vi "LoadData.vi"(8 "error in (no error)":errorcluster, 11 "AllData In":T1 {"FlukeData"."DataAnalysisArray"."TimeStamp" format="%^<%.3X\n%x>T"; "FlukeData"."ModelDataArray"."FREQUENCY" format="%#_6f"; "FlukeData"."ModelDataArray"."TimeStamp" format="%^<%.3X\n%x>T"; "FlukeData"."PMUDataArray"."FREQUENCY" format="%#_6f"; "FlukeData"."PMUDataArray"."TimeStamp" format="%^<%.3X\n%x>T"; "NISTData"."DataAnlysisArray"."Time" format="%.6f"; "NISTData"."DataAnlysisArray"."TimeStamp" format="%^<%.3X\n%x>T"; "NISTData"."DUTDataArray"."TimeStamp" format="%^<%.3X\n%x>T"; "NISTData"."DUTDataArray"."Time" format="%.6f"; "NISTData"."NIDataArray"."TimeStamp" format="%^<%.3X\n%x>T"; "NISTData"."NIDataArray"."Time" format="%.6f"}) -> (0 "error out":errorcluster, 3 "AllData Out":T1 {"FlukeData"."DataAnalysisArray"."TimeStamp" format="%^<%.3X\n%x>T"; "FlukeData"."ModelDataArray"."FREQUENCY" format="%#_6f"; "FlukeData"."ModelDataArray"."TimeStamp" format="%^<%.3X\n%x>T"; "FlukeData"."PMUDataArray"."FREQUENCY" format="%#_6f"; "FlukeData"."PMUDataArray"."TimeStamp" format="%^<%.3X\n%x>T"; "NISTData"."DataAnlysisArray"."Time" format="%.6f"; "NISTData"."DataAnlysisArray"."TimeStamp" format="%^<%.3X\n%x>T"; "NISTData"."DUTDataArray"."TimeStamp" format="%^<%.3X\n%x>T"; "NISTData"."DUTDataArray"."Time" format="%.6f"; "NISTData"."NIDataArray"."TimeStamp" format="%^<%.3X\n%x>T"; "NISTData"."NIDataArray"."Time" format="%.6f"})   [LabVIEW 2014]
uses:
  typedefs/Alldata.ctl
  typedefs/NISTData.ctl
  typedefs/NIDataArray.ctl
  typedefs/NIData.ctl
  typedefs/PhasorRectangular.ctl
  typedefs/DUTData.ctl
  typedefs/NICalcAnalysis.ctl
  typedefs/CalcPhasorError.ctl
  typedefs/PlotDataArrays.ctl
  typedefs/PmuRawDataCluster.ctl
  typedefs/CalcAnalysis.ctl
  typedefs/ePathsAction.ctl
  Fluke(lib)/Fluke(lib).lvlib
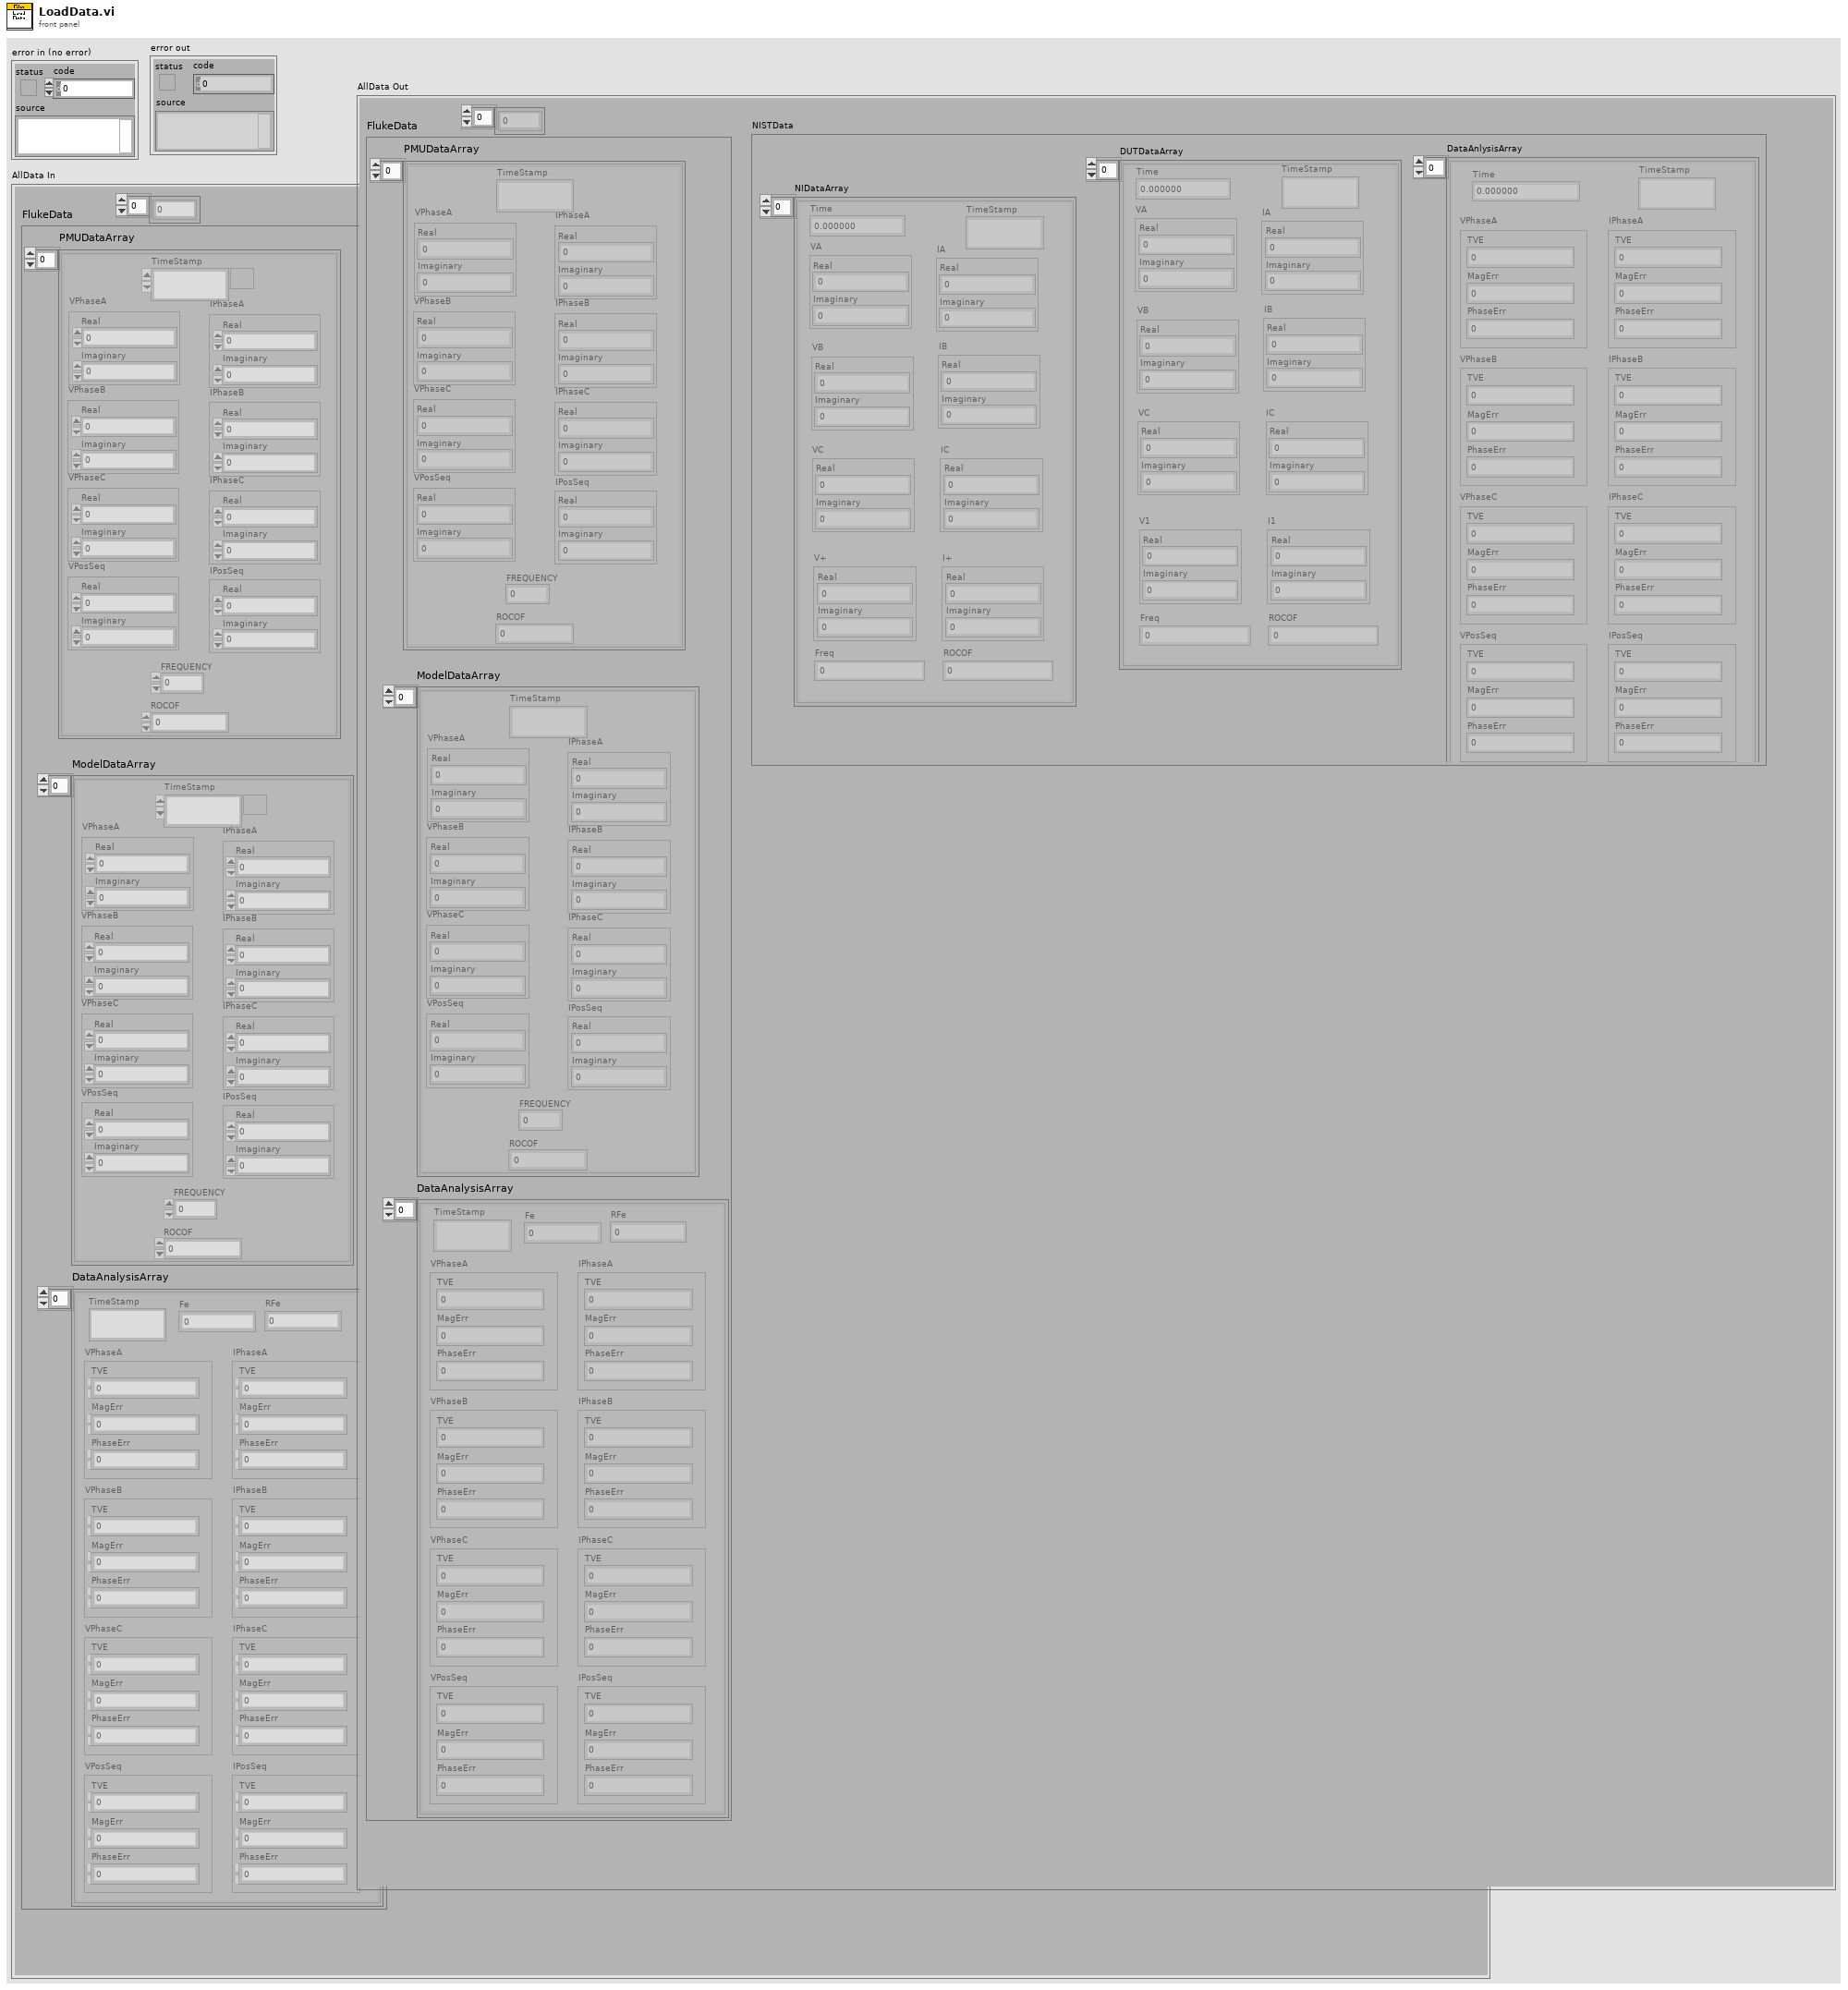
[diagram p1: front panel]
types:
  T1 = typedef "Alldata.ctl" = cluster{"NISTData":T2, "FlukeData":T9, "Params":dbl[]}
  T2 = typedef "NISTData.ctl" = cluster{"NIDataArray":T3, "DUTDataArray":T6[], "DataAnlysisArray":T7[]}
  T3 = typedef "NIDataArray.ctl" = T4[]
  T4 = typedef "NIData.ctl" = cluster{"Time":dbl, "VA":T5, "VB":T5, "VC":T5, "V+":T5, "IA":T5, "IB":T5, "IC":T5, "I+":T5, "Freq":dbl, "ROCOF":dbl, "TimeStamp":timestamp}
  T5 = typedef "PhasorRectangular.ctl" = cluster{"Real":dbl, "Imaginary":dbl}
  T6 = typedef "DUTData.ctl" = cluster{"Time":dbl, "VA":T5, "VB":T5, "VC":T5, "V1":T5, "IA":T5, "IB":T5, "IC":T5, "I1":T5, "Freq":dbl, "ROCOF":dbl, "TimeStamp":timestamp}
  T7 = typedef "NICalcAnalysis.ctl" = cluster{"Time":dbl, "VPhaseA":T8, "VPhaseB":T8, "VPhaseC":T8, "VPosSeq":T8, "IPhaseA":T8, "IPhaseB":T8, "IPhaseC":T8, "IPosSeq":T8, "Fe":dbl, "RFe":dbl, "TimeStamp":timestamp}
  T8 = typedef "CalcPhasorError.ctl" = cluster{"TVE":dbl, "MagErr":dbl, "PhaseErr":dbl}
  T9 = typedef "PlotDataArrays.ctl" = cluster{"PMUDataArray":T10[], "ModelDataArray":T10[], "DataAnalysisArray":T11[]}
  T10 = typedef "PmuRawDataCluster.ctl" = cluster{"TimeStamp":timestamp, "VPhaseA":T5, "VPhaseB":T5, "VPhaseC":T5, "VPosSeq":T5, "IPhaseA":T5, "IPhaseB":T5, "IPhaseC":T5, "IPosSeq":T5, "FREQUENCY":dbl, "ROCOF":sgl}
  T11 = typedef "CalcAnalysis.ctl" = cluster{"TimeStamp":timestamp, "VPhaseA":T8, "VPhaseB":T8, "VPhaseC":T8, "VPosSeq":T8, "IPhaseA":T8, "IPhaseB":T8, "IPhaseC":T8, "IPosSeq":T8, "Fe":dbl, "RFe":dbl}
  T12 = typedef "ePathsAction.ctl" = enum16{"Set", "Get", "Load", "Save", "Default", "Exit"}
  T13 = typedef "Paths.ctl" = cluster{"BasePath":path, "CutPath":path, "LastCutPath":path, "CCSPath":path, "LastCCSPath":path, "ResultsPath":path}
  T14 = typedef "Fluke(lib).lvlib/TestParams.ctl" = cluster{"TestType":dbl, "F0":dbl, "Fs":dbl, "Fin":dbl, "dF":dbl, "Pin":dbl, "Iin":dbl, "Ki":dbl, "Vin":dbl, "Kv":dbl, "Fh":dbl, "Kh":dbl, "Ph":dbl, "Fi":dbl, "Kintr":dbl, "Pi":dbl, "Fx":dbl, "Kx":dbl, "Px":dbl, "Fa":dbl, "Ka":dbl, "Pa":dbl, "Sec":dbl, "Reports":dbl, "Frac":dbl, "Divisor":dbl}
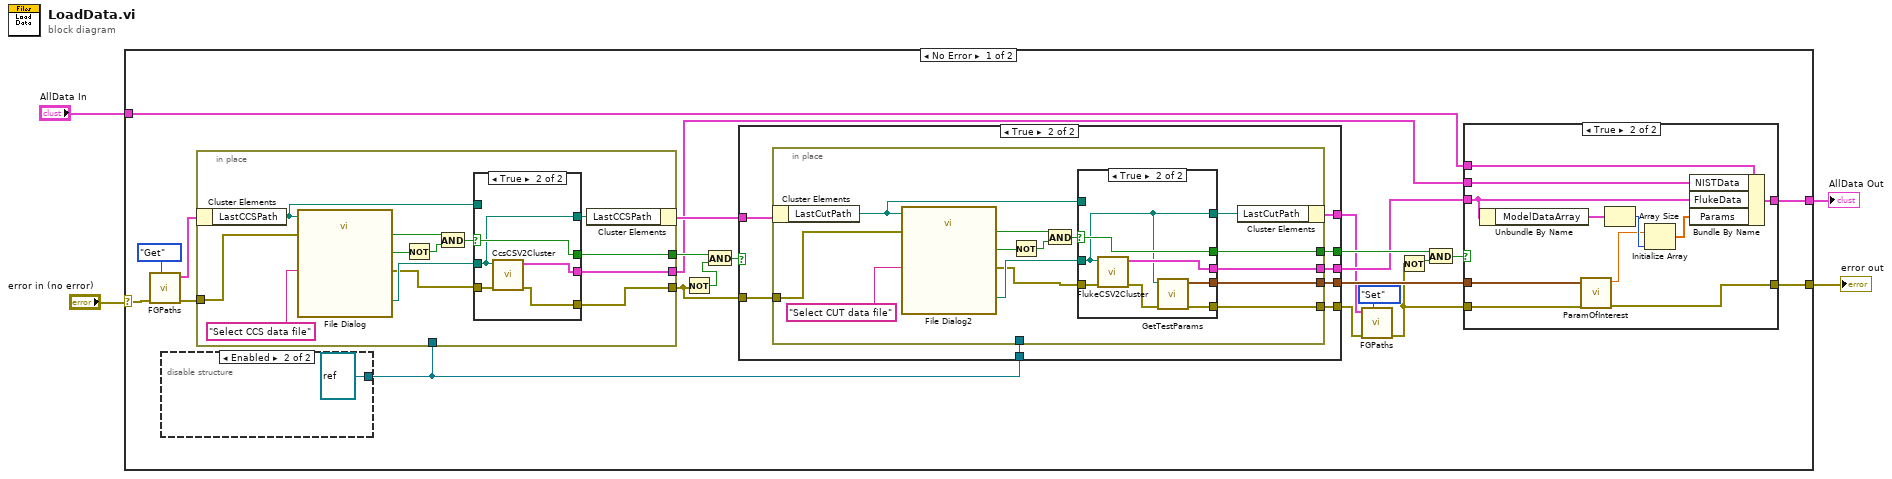
[diagram p0: block diagram]
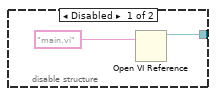
[diagram p2: hidden frame]
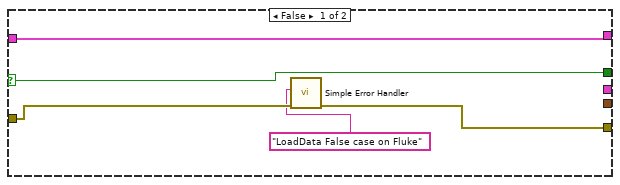
[diagram p4: hidden frame]
diagram:
  n1 = case shown="No Error" "error in (no error)" {
    selector: "error in (no error)" -> [w27 w103]
    tunnel: [w12 w103] -> w3
    tunnel: "AllData In" -> [w14 w102]
    tunnel: [w13 w102] -> w1
    frame No Error {
      n2 = call "FGPaths.vi"("ePathsAction"=ePathsAction."Get", "error in (no error)"=w27) -> ("error out"=w25:errorcluster, "PathsOut"=w11:T13)  [unwired: 8 in]
      n3 = disable-structure shown="Enabled" {
        disable-tunnel: [w28 refnum<vi> refnum ("vi reference")] -> w10
        frame Disabled {
          n4 = Open VI Reference(vi path="main.vi") -> (vi reference=w28:refnum<vi>)  [unwired: 5 in, 1 out]
        }
        frame Enabled {
        }
      }
      n5 = in-place {
        in-place-border: w25 -> [w93]
        in-place-border: [w84] -> w22
        in-place-border: [w83] -> w16
        in-place-border: [w81] -> w24
        in-place-border: w10 -> [_]
        n6 = in-place-cluster #1(w11) -> ("LastCCSPath"=w87:path)
        n7 = call "File Dialog"("start path"=w87, "prompt"="Select CCS data file", "error in"=w93) -> ("selected path"=w85:path, "exists"=w90:bool, "cancelled"=w88:bool, "error out"=w82:errorcluster)  [unwired: 9 in]
        n8 = Not(x=w88) -> (.not. x?=w89:bool)
        n9 = And(x=w90, y=w89) -> (x .and. y?=w91:bool)
        n10 = case shown="True" w91 {
          selector: w91 -> [w94 w100]
          tunnel: [w96 w98] -> w86
          tunnel: w87 -> [w96 _]
          tunnel: w85 -> [_ w98]
          tunnel: w82 -> [w95 w101]
          tunnel: [w95 w97] -> w81
          tunnel: [w94 w100] -> w84
          tunnel: [_ w99] -> w83
          frame False {
          }
          frame True {
            n11 = call "CcsCSV2Cluster.vi"("error in (no error)"=w101, "CCSPath"=w98) -> ("error out"=w97:errorcluster, "AllDataArrays"=w99:T2)  [unwired: 8 in]
          }
        }
        n12 = in-place-cluster #1("LastCCSPath"=w86) -> (w20:T13)
      }
      n13 = Not(x=w24) -> (.not. x?=w21:bool)
      n14 = And(x=w22, y=w21) -> (x .and. y?=w23:bool)
      n15 = case shown="True" w23 {
        selector: w23 -> [w48 _]
        tunnel: w24 -> [w47 w56]
        tunnel: w20 -> [w44 w55]
        tunnel: [w48 w54] -> w18
        tunnel: [w46 w53] -> w7
        tunnel: [_ w52] -> w15
        tunnel: w10 -> [_ w51]
        tunnel: [_ w50] -> w9
        tunnel: [w44 w49] -> w6
        frame False {
          n16 = call <vilib>:"Simple Error Handler.vi"("error source (\" \")"="LoadData False case on Fluke", "error in (no error)"=w47) -> ("error out"=w46:errorcluster)  [unwired: 3 in, 4 out]
        }
        frame True {
          n17 = in-place {
            in-place-border: w56 -> [w70]
            in-place-border: [w61] -> w54
            in-place-border: [w60] -> w52
            in-place-border: [w58] -> w53
            in-place-border: w51 -> [_]
            in-place-border: [w57] -> w50
            n18 = in-place-cluster #2(w55) -> ("LastCutPath"=w64:path)
            n19 = call "File Dialog2"("start path"=w64, "prompt"="Select CUT data file", "error in"=w70) -> ("selected path"=w62:path, "exists"=w67:bool, "cancelled"=w65:bool, "error out"=w59:errorcluster)  [unwired: 9 in]
            n20 = Not(x=w65) -> (.not. x?=w66:bool)
            n21 = And(x=w67, y=w66) -> (x .and. y?=w68:bool)
            n22 = case shown="True" w68 {
              selector: w68 -> [w71 w79]
              tunnel: [w73 w75] -> w63
              tunnel: w64 -> [w73 _]
              tunnel: w62 -> [_ w75]
              tunnel: w59 -> [w72 w80]
              tunnel: [w72 w76] -> w58
              tunnel: [w71 w79] -> w61
              tunnel: [_ w78] -> w60
              tunnel: [_ w74] -> w57
              frame False {
              }
              frame True {
                n23 = call "FlukeCSV2Cluster.vi"("error in (no error)"=w80, "FlukePath"=w75) -> ("error out"=w77:errorcluster, "AllDataArrays"=w78:T9)  [unwired: 8 in]
                n24 = call "GetTestParams.vi"("error in (no error)"=w77, "RawData Filename"=w75) -> ("error out"=w76:errorcluster, "TestParams"=w74:T14)  [unwired: 8 in]
              }
            }
            n25 = in-place-cluster #2("LastCutPath"=w63) -> (w49:T13)
          }
        }
      }
      n26 = call "FGPaths.vi"("ePathsAction"=ePathsAction."Set", "error in (no error)"=w7, "PathsIn"=w6) -> ("error out"=w8:errorcluster)  [unwired: 7 in, 1 out]
      n27 = Not(x=w8) -> (.not. x?=w17:bool)
      n28 = And(x=w18, y=w17) -> (x .and. y?=w19:bool)
      n29 = case shown="True" w19 {
        tunnel: w8 -> [w31 w40]
        tunnel: w16 -> [_ w43]
        tunnel: w15 -> [_ w37]
        tunnel: w14 -> [w32 w42]
        tunnel: [w32 w41] -> w13
        tunnel: [w31 w39] -> w12
        tunnel: w9 -> [_ w38]
        frame False {
        }
        frame True {
          n30 = Unbundle By Name(w37) -> ("ModelDataArray"=w36:T10[])
          n31 = call "ParamOfInterest.vi"("error in (no error)"=w40, "TestParams"=w38) -> ("error out"=w39:errorcluster, "Param"=w34:dbl)  [unwired: 8 in]
          n32 = Array Size(array=w36) -> (size(s)=w35:i32)
          n33 = Initialize Array(w34, w35) -> (w33:dbl[])
          n34 = Bundle By Name(cluster=w42, "NISTData"=w43, "FlukeData"=w37, "Params"=w33) -> (w41:T1)
        }
      }
    }
    frame Error {
    }
  }
  "error out" <- w3
  "AllData Out" <- w1
